vi "Graph Page.vi"() -> ()   [LabVIEW 2020, in "3D Plot.lvclass"]
uses:
  <vilib>/Math Plots/3D Math Plots/3D Plot/3D Plot/3D Plot.lvclass
  <vilib>/Math Plots/3D Math Plots/3D Plot/3D Plot/Typedef/Graph Property.ctl
  <vilib>/Math Plots/3D Math Plots/3D Plot/3D Plot/Typedef/General Property.ctl
  <vilib>/Math Plots/3D Math Plots/3D Plot/3D Plot/Typedef/View Property.ctl
  <vilib>/Math Plots/3D Math Plots/3D Plot/3D Plot/Typedef/Grid Plane.ctl
  <vilib>/Math Plots/3D Math Plots/3D Plot/3D Plot/Typedef/Dialog State.ctl
  <vilib>/Math Plots/3D Math Plots/3D Plot/3D Plot/Typedef/Temp Scene State.ctl
  <vilib>/Math Plots/3D Math Plots/3D Plot/3D Plot/Typedef/Temp Scene Property Action.ctl
panel:
  in  "Grid Frame Color":u32(colorbox) caption="Grid frame color"
  in  "Y-Z Plane Visible":bool caption="Y-Z plane visible"
  in  "X-Z Plane Visible":bool caption="X-Z plane visible"
  in  "X-Y Plane Visible":bool caption="X-Y plane visible"
  in  "Grid Antialiasing":bool caption="Grid antialiasing"
  in  "Distance":sgl(slide) scale=0.0..20.0
  in  "Latitude":sgl(slide) min=0 max=360 scale=0.0..360.0
  in  "Longitude":sgl(slide) min=0 max=360 scale=0.0..360.0
  in  "View Projection":u16(ring) caption="View projection" items=["Orthographic", "Perspective"]
  in  "View direction":T1(radio)
  in  "Clip Data":bool caption="Clip data"
  in  "Fast Draw":bool caption="Fast draw"
  in  "Background Color":u32(colorbox) caption="Background color"
  in  "Event Registration":refnum<event-registration>
  out "Graph Property Out":T2
  in  "Graph Property In":T2
  # "Graph"
  # "General Setting"
  # "Grid Plane"
  # "View Direction"
  # "User Defined View"
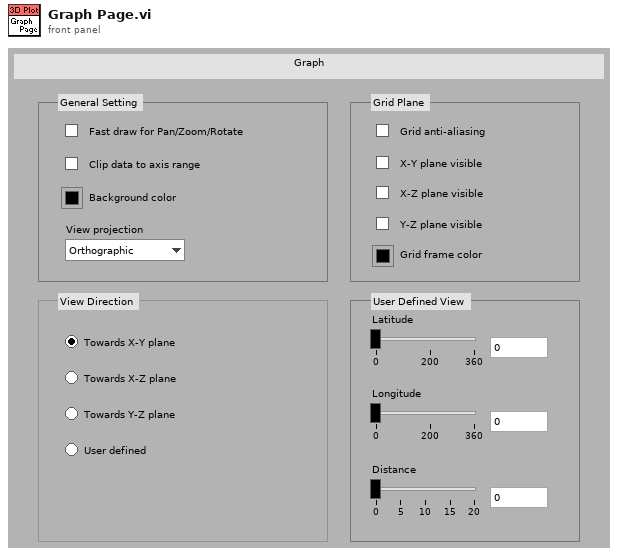
[diagram p1: front panel]
types:
  T1 = enum32{"Towards X-Y Plane", "Towards Y-Z Plane", "Towards X-Z Plane", "User Defined"}
  T2 = typedef "3D Plot.lvclass/Graph Property.ctl" = cluster{"General Property":T3, "View Property":T4, "Grid Plane":T5}
  T3 = typedef "3D Plot.lvclass/General Property.ctl" = cluster{"Plot Area Color":u32, "Fast Draw?":bool, "Clip Data?":bool}
  T4 = typedef "3D Plot.lvclass/View Property.ctl" = cluster{"Projection Mode":enum16{"Orthographic", "Perspective"}, "View Direction":enum32{"Towards X-Y Plane", "Towards X-Z Plane", "Towards Y-Z Plane", "User Defined"}, "User Defined View Direction":cluster{"View Latitude":sgl, "View Longitude":sgl, "View Distance":sgl}}
  T5 = typedef "3D Plot.lvclass/Grid Plane.ctl" = cluster{"Grid Plane Visible":cluster{"Draw Grid Plane X-Y":bool, "Draw Grid Plane Y-Z":bool, "Draw Grid Plane X-Z":bool}, "Grid Antialiasing":bool, "Grid Frame Color":u32}
  T6 = typedef "3D Plot.lvclass/Dialog State.ctl" = enum16{"Initialize", "Read Porperty", "Write Property", "Idle", "Exit"}
  T7 = typedef "3D Plot.lvclass/Temp Scene Property Action.ctl" = enum16{"Graph Property", "Light Property", "Axis Property", "Value Pair Property", "Format Property", "Cursor Property", "Plot Specific Property"}
  T8 = typedef "3D Plot.lvclass/Temp Scene State.ctl" = enum16{"Create", "Update Scene", "Get Plot Representation", "Destory"}
  T9 = enum32{"Towards X-Y Plane", "Towards X-Z Plane", "Towards Y-Z Plane", "User Defined"}
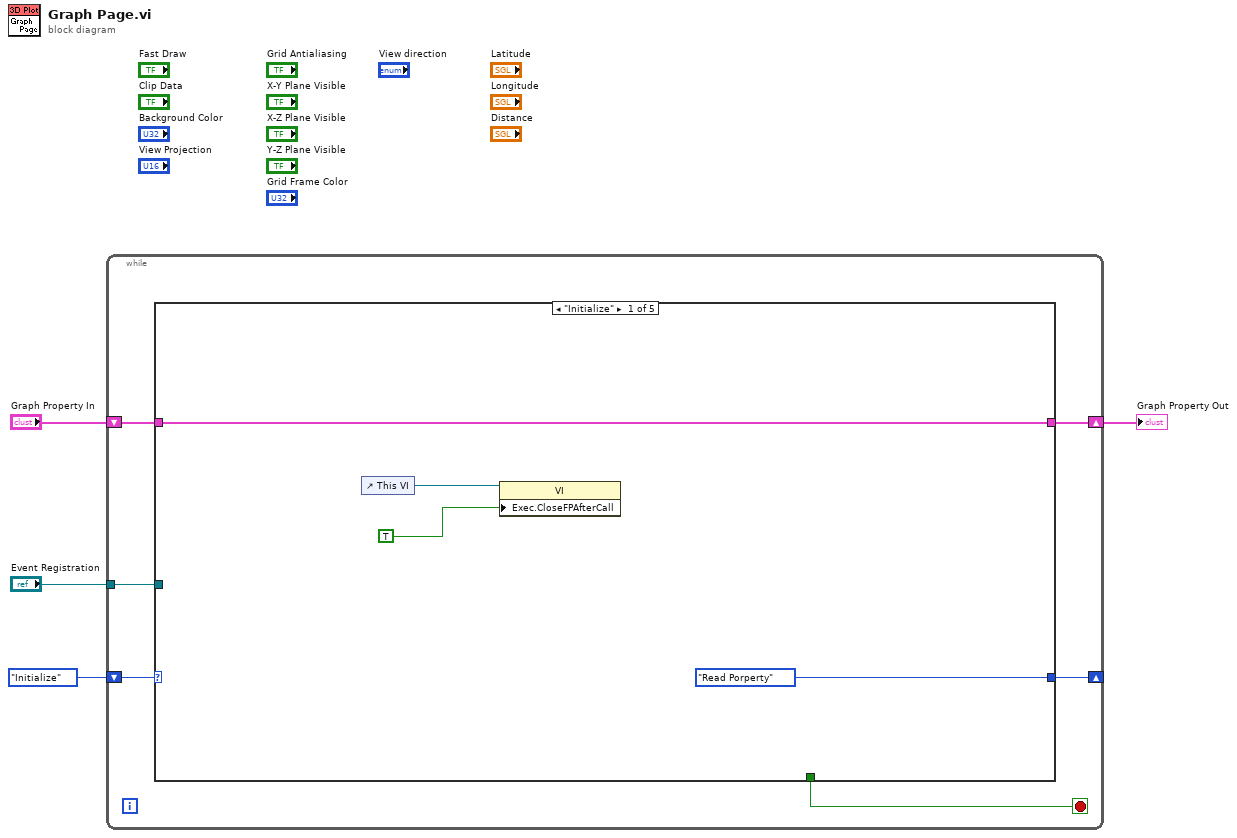
[diagram p0: block diagram]
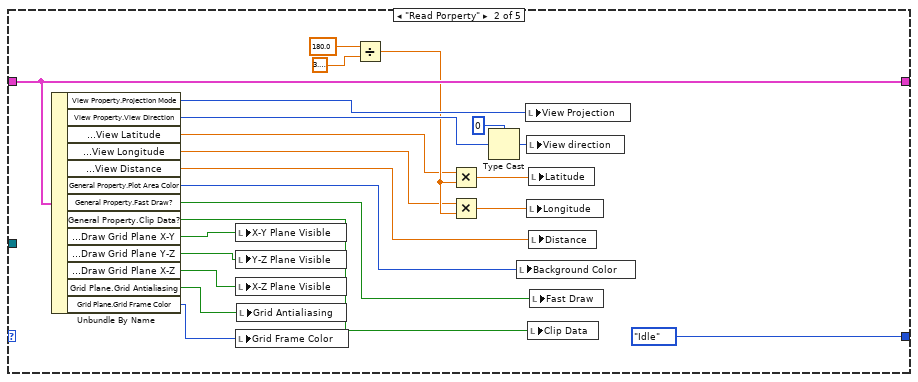
[diagram p2: hidden frame]
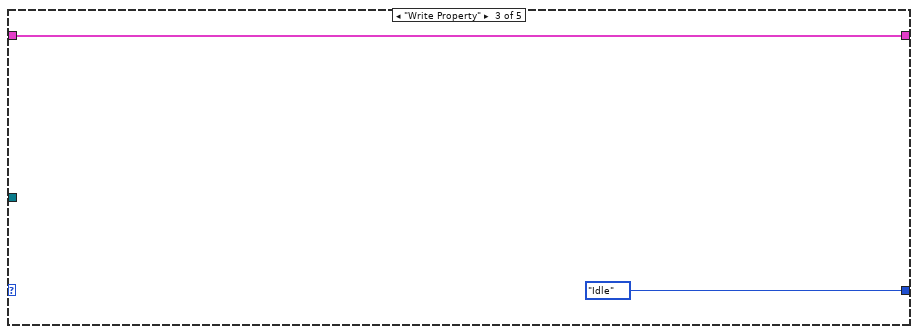
[diagram p3: hidden frame]
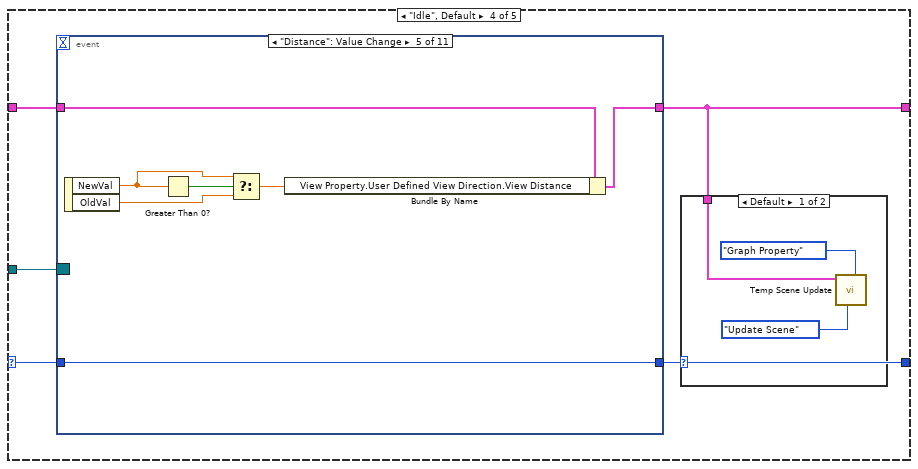
[diagram p4: hidden frame]
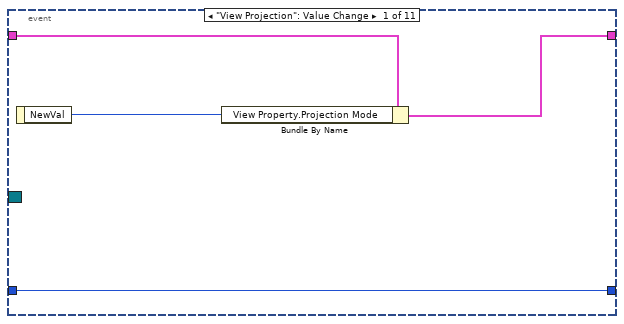
[diagram p6: hidden frame]
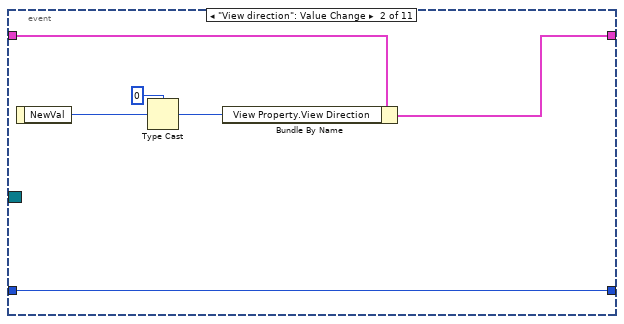
[diagram p7: hidden frame]
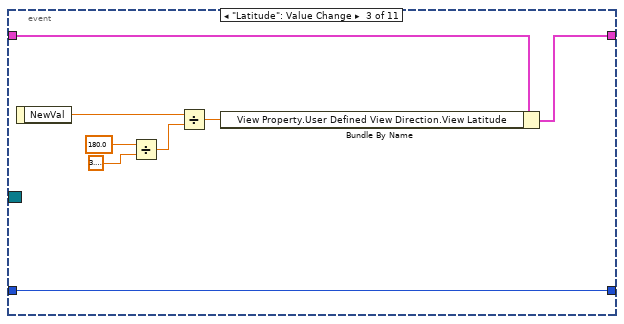
[diagram p8: hidden frame]
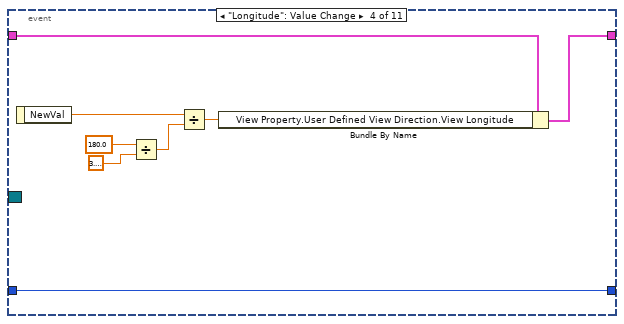
[diagram p9: hidden frame]
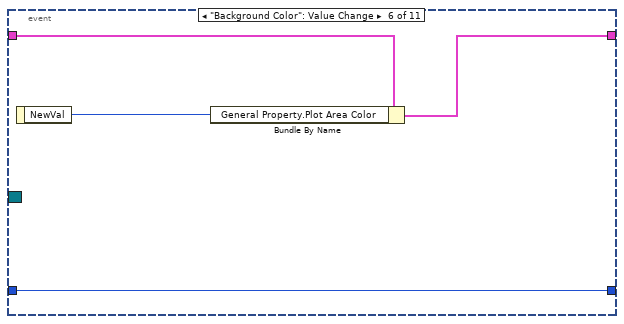
[diagram p10: hidden frame]
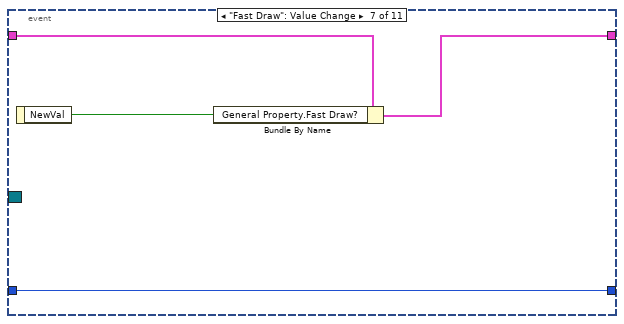
[diagram p11: hidden frame]
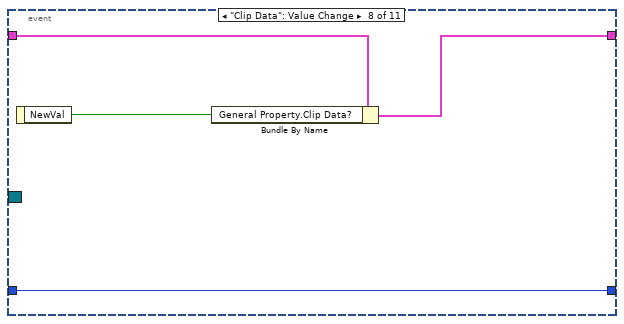
[diagram p12: hidden frame]
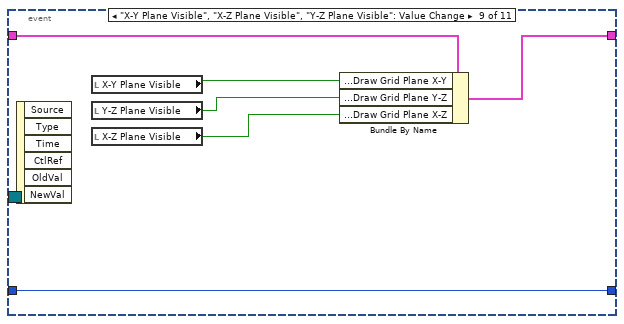
[diagram p13: hidden frame]
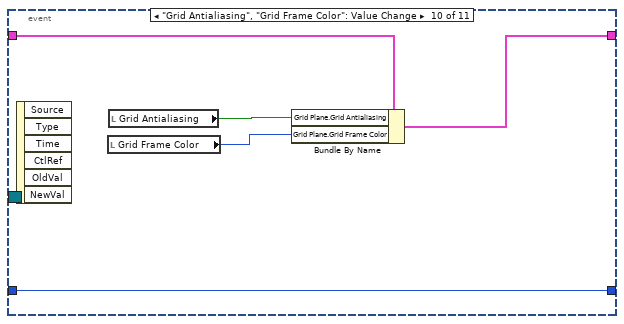
[diagram p14: hidden frame]
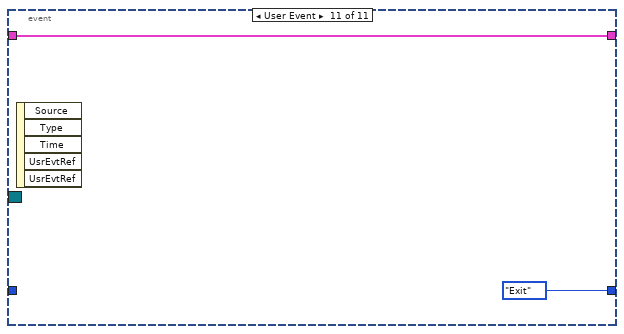
[diagram p15: hidden frame]
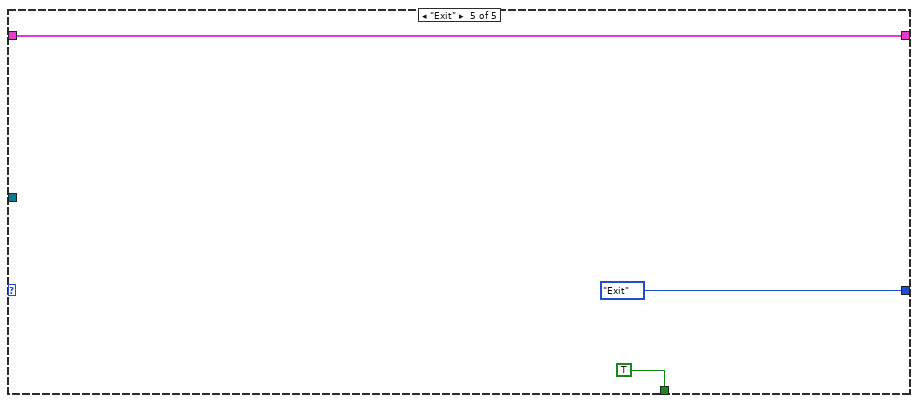
[diagram p16: hidden frame]
diagram:
  n1 = while {
    shift-right: [w9] -> w3
    shift-left: "Graph Property In" -> [w10]
    shift-right: [w5] -> _
    shift-left: Dialog_State."Initialize" ("Enum") -> [w6]
    tunnel: "Event Registration" -> [w7]
    stop <- w8 stop-if-true
    n2 = case shown="\"Initialize\"" w6 {
      selector: w6 -> [_ _ _ w41 _]
      tunnel: w10 -> [w14 w36 w37 w43 w105]
      tunnel: [w14 w36 w37 w40 w105] -> w9
      tunnel: [Dialog_State."Read Porperty" ("Enum") Dialog_State."Idle" Dialog_State."Idle" w39 Dialog_State."Exit"] -> w5
      tunnel: [_ _ _ _ TRUE] -> w8
      tunnel: w7 -> [_ _ _ w42 _]
      frame "Initialize" {
        n3 = control-ref of="This VI"() -> (w13:refnum<vi>)
        n4 = property class="VI"(reference=w13, "Exec.CloseFPAfterCall"=TRUE ("Execution:Close After Call")) -> ()  [unwired: 1 in, 2 out]
      }
      frame "Read Porperty" {
        n5 = Unbundle By Name(w36) -> ("View Property.Projection Mode"=w35:enum16{"Orthographic", "Perspective"}, "View Property.View Direction"=w30:T9, "View Property.User Defined View Direction.View Latitude"=w22:sgl, "View Property.User Defined View Direction.View Longitude"=w21:sgl, "View Property.User Defined View Direction.View Distance"=w15:sgl, "General Property.Plot Area Color"=w34:u32, "General Property.Fast Draw?"=w33:bool, "General Property.Clip Data?"=w32:bool, "Grid Plane.Grid Plane Visible.Draw Grid Plane X-Y"=w20:bool, "Grid Plane.Grid Plane Visible.Draw Grid Plane Y-Z"=w19:bool, "Grid Plane.Grid Plane Visible.Draw Grid Plane X-Z"=w18:bool, "Grid Plane.Grid Antialiasing"=w17:bool, "Grid Plane.Grid Frame Color"=w16:u32)
        n6 = local write "X-Y Plane Visible"(w20) -> ()
        n7 = local write "Y-Z Plane Visible"(w19) -> ()
        n8 = local write "X-Z Plane Visible"(w18) -> ()
        n9 = local write "Grid Frame Color"(w16) -> ()
        n10 = local write "Grid Antialiasing"(w17) -> ()
        n11 = Divide(x=sgl 180.0, y=sgl 3.1415927) -> (x/y=w27:sgl)
        n12 = Multiply(x=w22, y=w27) -> (x*y=w24:sgl)
        n13 = Multiply(x=w21, y=w27) -> (x*y=w23:sgl)
        n14 = Type Cast(type=u32 0, x=w30) -> (*(type *) &x=w29:u32)
        n15 = local write "Background Color"(w34) -> ()
        n16 = local write "View Projection"(w35) -> ()
        n17 = local write "View direction"(w29) -> ()
        n18 = local write "Longitude"(w23) -> ()
        n19 = local write "Clip Data"(w32) -> ()
        n20 = local write "Latitude"(w24) -> ()
        n21 = local write "Distance"(w15) -> ()
        n22 = local write "Fast Draw"(w33) -> ()
      }
      frame "Write Property" {
      }
      frame "Idle", Default {
        n23 = event shown="[4] \"Distance\": Value Change" {
          selector: w42 -> [_ _ _ _ _ _ _ _ _ _ _]
          dyn-events: _ -> [_ _ _ _ _ _ _ _ _ _ _]
          timeout: _ -> [_ _ _ _ _ _ _ _ _ _ _]
          tunnel: w43 -> [w50 w56 w64 w72 w79 w83 w87 w91 w97 w102 w104]
          tunnel: [w49 w55 w63 w71 w78 w82 w86 w90 w96 w101 w104] -> w40
          tunnel: [w47 w51 w62 w70 w77 w80 w84 w88 w92 w98 Dialog_State."Exit"] -> w39
          tunnel: w41 -> [w47 w51 w62 w70 w77 w80 w84 w88 w92 w98 _]
          event "View Projection": Value Change {
            n24 = event-data() -> ("NewVal"=w48:u16)  [unwired: 1 out]
            n25 = Bundle By Name(cluster=w50, "View Property.Projection Mode"=w48) -> (w49:T2)
          }
          event "View direction": Value Change {
            n26 = event-data() -> ("NewVal"=w53:T1)  [unwired: 1 out]
            n27 = Type Cast(type=u32 0, x=w53) -> (*(type *) &x=w52:u32)
            n28 = Bundle By Name(cluster=w56, "View Property.View Direction"=w52) -> (w55:T2)
          }
          event "Latitude": Value Change {
            n29 = event-data() -> ("NewVal"=w58:sgl)  [unwired: 1 out]
            n30 = Divide(x=sgl 180.0, y=sgl 3.1415927) -> (x/y=w59:sgl)
            n31 = Divide(x=w58, y=w59) -> (x/y=w57:sgl)
            n32 = Bundle By Name(cluster=w64, "View Property.User Defined View Direction.View Latitude"=w57) -> (w63:T2)
          }
          event "Longitude": Value Change {
            n33 = event-data() -> ("NewVal"=w66:sgl)  [unwired: 1 out]
            n34 = Divide(x=sgl 180.0, y=sgl 3.1415927) -> (x/y=w67:sgl)
            n35 = Divide(x=w66, y=w67) -> (x/y=w65:sgl)
            n36 = Bundle By Name(cluster=w72, "View Property.User Defined View Direction.View Longitude"=w65) -> (w71:T2)
          }
          event "Distance": Value Change {
            n37 = event-data() -> ("NewVal"=w75:sgl, "OldVal"=w74:sgl)  [unwired: 1 out]
            n38 = Greater Than 0?(x=w75) -> (x > 0?=w76:bool)
            n39 = Select(t=w75, s=w76, f=w74) -> (s? t:f=w73:sgl)
            n40 = Bundle By Name(cluster=w79, "View Property.User Defined View Direction.View Distance"=w73) -> (w78:T2)
          }
          event "Background Color": Value Change {
            n41 = event-data() -> ("NewVal"=w81:u32)  [unwired: 1 out]
            n42 = Bundle By Name(cluster=w83, "General Property.Plot Area Color"=w81) -> (w82:T2)
          }
          event "Fast Draw": Value Change {
            n43 = event-data() -> ("NewVal"=w85:bool)  [unwired: 1 out]
            n44 = Bundle By Name(cluster=w87, "General Property.Fast Draw?"=w85) -> (w86:T2)
          }
          event "Clip Data": Value Change {
            n45 = event-data() -> ("NewVal"=w89:bool)  [unwired: 1 out]
            n46 = Bundle By Name(cluster=w91, "General Property.Clip Data?"=w89) -> (w90:T2)
          }
          event "X-Y Plane Visible", "X-Z Plane Visible", "Y-Z Plane Visible": Value Change {
            n47 = event-data() -> ()  [unwired: 7 out]
            n48 = local read "X-Y Plane Visible"() -> (w95:bool)
            n49 = local read "Y-Z Plane Visible"() -> (w94:bool)
            n50 = local read "X-Z Plane Visible"() -> (w93:bool)
            n51 = Bundle By Name(cluster=w97, "Grid Plane.Grid Plane Visible.Draw Grid Plane X-Y"=w95, "Grid Plane.Grid Plane Visible.Draw Grid Plane Y-Z"=w94, "Grid Plane.Grid Plane Visible.Draw Grid Plane X-Z"=w93) -> (w96:T2)
          }
          event "Grid Antialiasing", "Grid Frame Color": Value Change {
            n52 = event-data() -> ()  [unwired: 7 out]
            n53 = local read "Grid Frame Color"() -> (w99:u32)
            n54 = local read "Grid Antialiasing"() -> (w100:bool)
            n55 = Bundle By Name(cluster=w102, "Grid Plane.Grid Antialiasing"=w100, "Grid Plane.Grid Frame Color"=w99) -> (w101:T2)
          }
          event User Event {
            n56 = event-data() -> ()  [unwired: 6 out]
          }
        }
        n57 = case shown="Default" w39 {
          tunnel: w40 -> [w46 _]
          frame Default {
            n58 = call <vilib>:"Temp Scene Update.vi"("Property Name"=Temp_Scene_Property_Action."Graph Property", "State"=Temp_Scene_State."Update Scene", "Property In"=w46) -> ()  [unwired: 3 in, 6 out]
          }
          frame "Exit" {
          }
        }
      }
      frame "Exit" {
      }
    }
  }
  "Graph Property Out" <- w3
